vi "WaitOccurance.vi"(1 "Occurrence Refnum":refnum<k4>) -> (0 "String Output":string)   [LabVIEW 2012]
panel:
  # "Waiting For Occurance...."
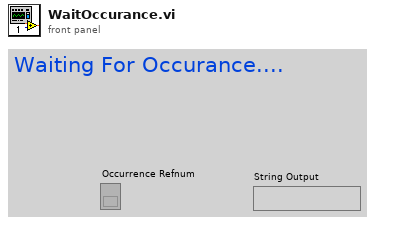
[diagram p1: front panel]
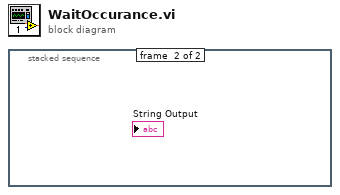
[diagram p0: block diagram]
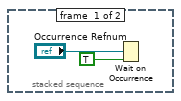
[diagram p2: hidden frame]
diagram:
  n1 = stacked-sequence "Sequence Structure" {
    frame #0 {
      n2 = Wait on Occurrence(1:TRUE ("ignore previous (T)"), 2:"Occurrence Refnum") -> ()  [unwired: 2 out]
    }
    frame #1 {
    }
  }
